vi "msg read from ARDUINO.vi"(8 "error in (read msg)":errorcluster, 11 "VISA Refnum in":refnum<visa-resource-name>) -> (1 "error out (read msg)":errorcluster, 2 "msg answer":string, 3 "VISA Refnum out":refnum<visa-resource-name>)   [LabVIEW 2018]
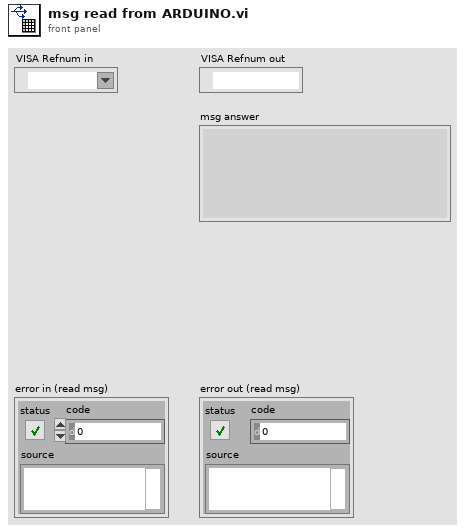
[diagram p1: front panel]
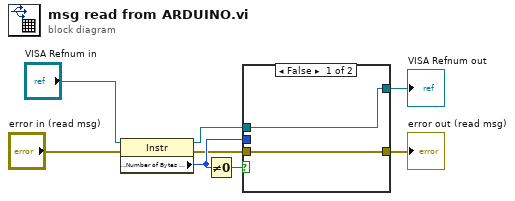
[diagram p0: block diagram]
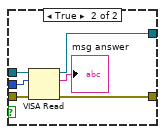
[diagram p2: hidden frame]
diagram:
  n1 = property class="Instr"(reference="VISA Refnum in", error in="error in (read msg)") -> (reference out=w2:refnum<visa-resource-name>, error out=w4:errorcluster, "Serial Settings:Number of Bytes at Serial Port"=w7:u32)
  n2 = Not Equal To 0?(x=w7) -> (x != 0?=w8:bool)
  n3 = case shown="False" w8 {
    tunnel: w7 -> [_ w16]
    tunnel: w2 -> [w10 w15]
    tunnel: w4 -> [w9 w14]
    tunnel: [w10 w12] -> w5
    tunnel: [w9 w11] -> w6
    frame False {
    }
    frame True {
      n4 = VISA Read(VISA resource name=w15, byte count=w16, error in (no error)=w14) -> (VISA resource name out=w12:refnum<visa-resource-name>, read buffer=→"msg answer":string, error out=w11:errorcluster)  [unwired: 1 out]
    }
  }
  "error out (read msg)" <- w6
  "VISA Refnum out" <- w5
